vi "e.gate HighSpeedPort Decode Buffer Variable Header Data.vi"(0 "Data in (binary)":u8[](array[numeric]), 1 "Configuration in":T1, 11 "error in (no error)":errorcluster) -> (3 "Configuration out":T1, 4 "Remaining Data out":u8[](array[numeric]), 15 "error out":errorcluster)   [LabVIEW 2016]
doc: "This VI is used to decode all channel related data from a UDBF coded stream to an array of channel data clusters in the configuration cluster."
uses:
  e.gate Configuration.ctl
  e.gate Channel Data.ctl
  e.gate Data Type.ctl
  e.gate Protocol Type.ctl
  e.gate Module  Data.ctl
  e.gateHSP_DLLhandle.ctl
panel:
  out "ChannelAdditionalDatLen 2":i32
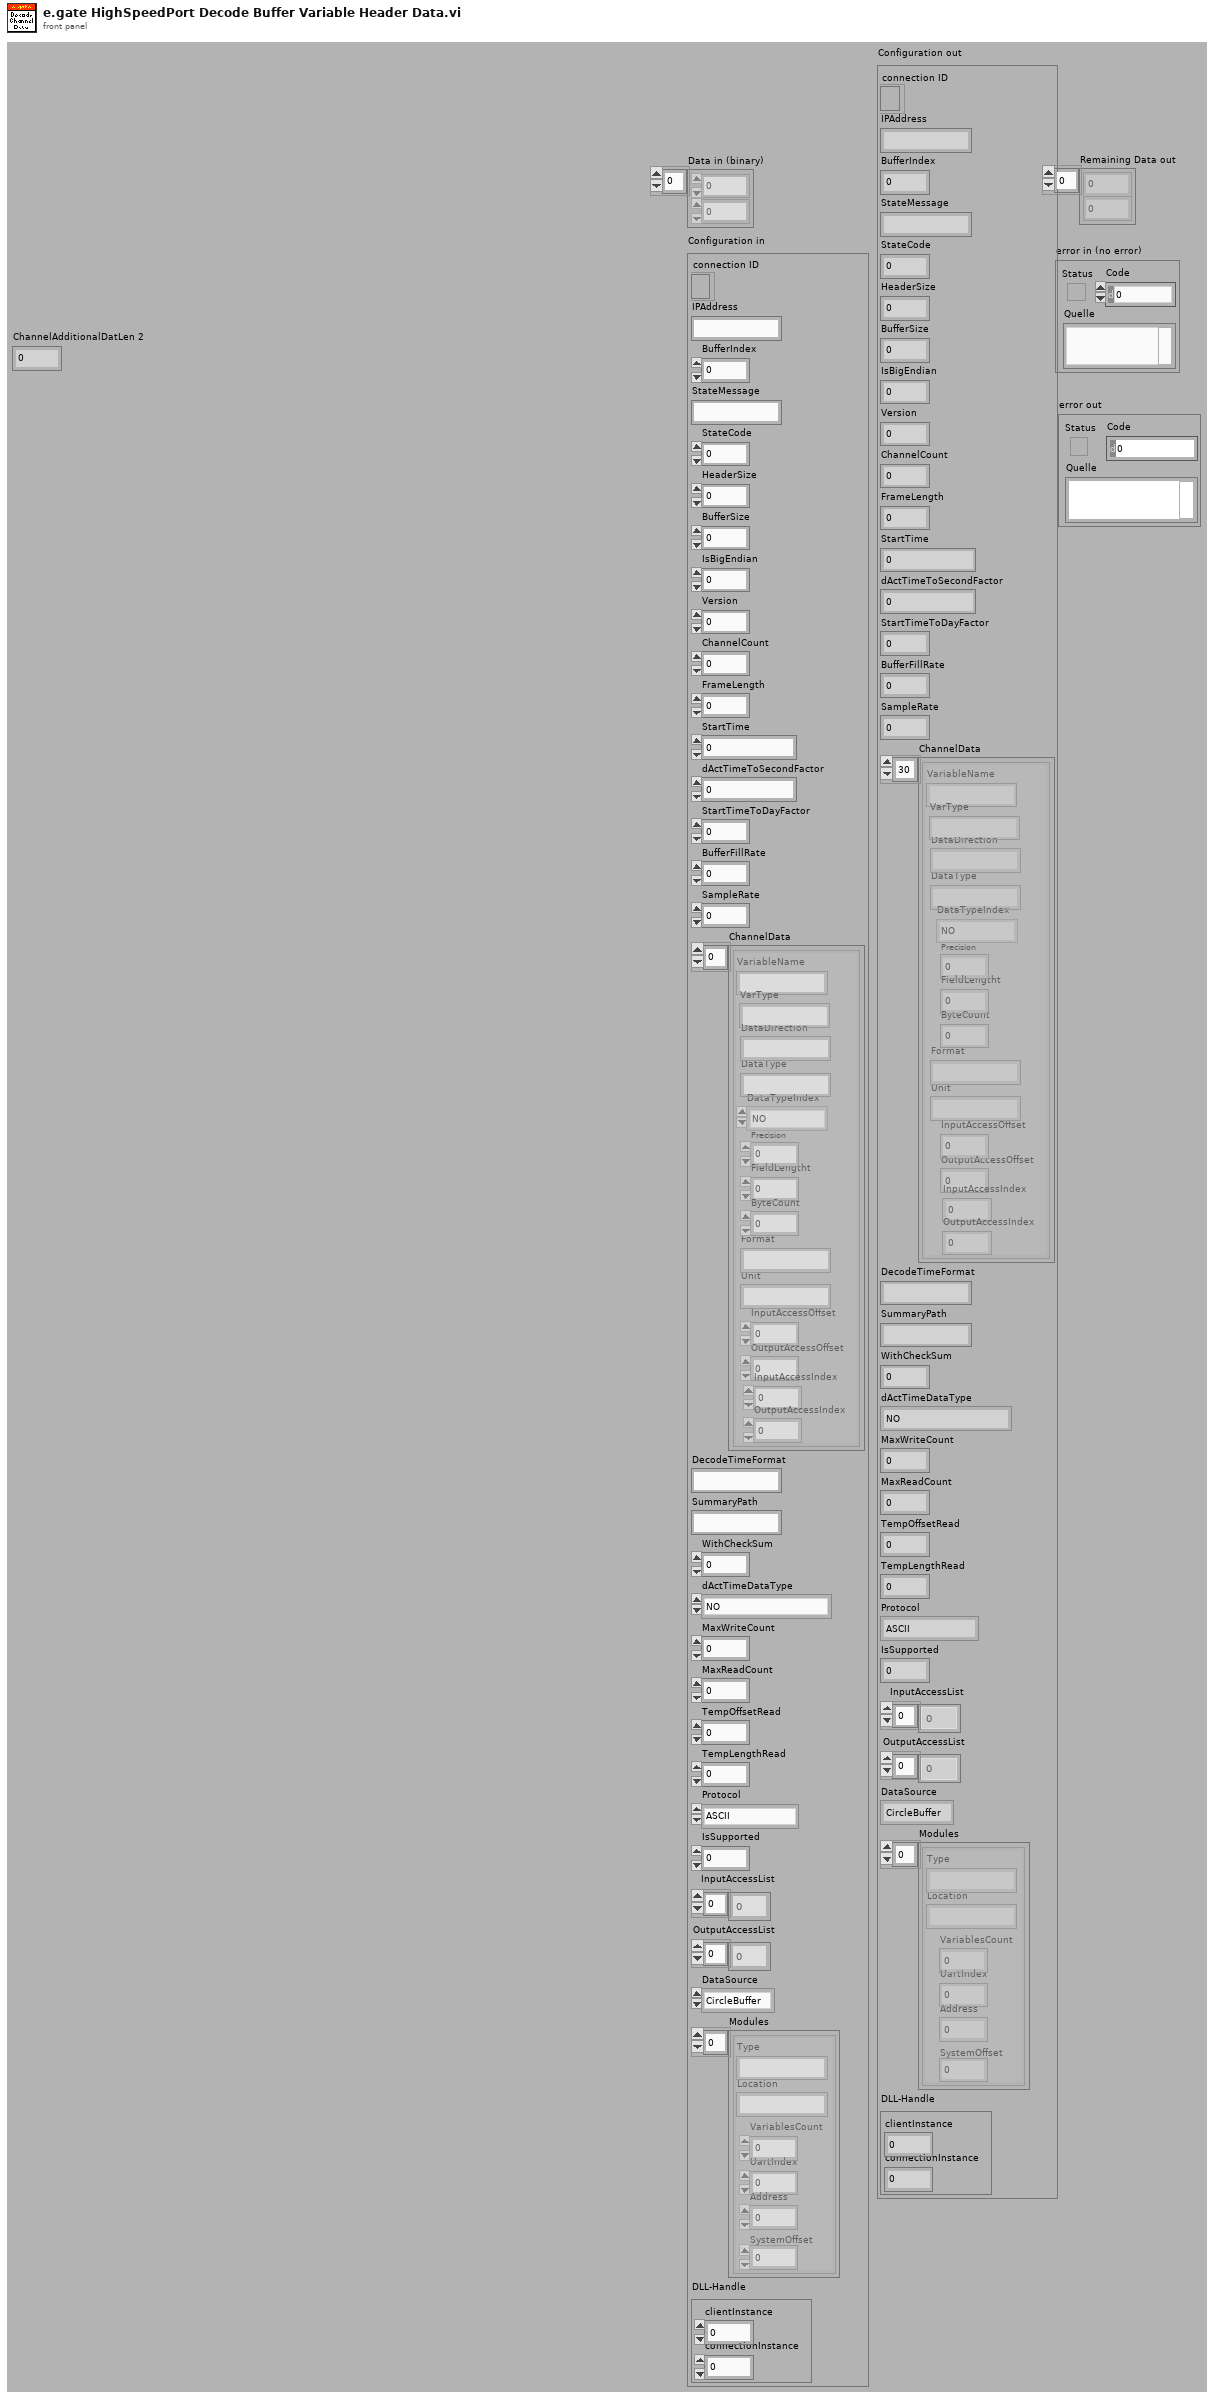
[diagram p1: front panel]
types:
  T1 = typedef "e.gate Configuration.ctl" = cluster{"connection ID":refnum<k5>, "IPAddress":string, "BufferIndex":i32, "StateMessage":string, "StateCode":i8, "HeaderSize":i32, "BufferSize":i32, "IsBigEndian":i32, "Version":i32, "ChannelCount":i32, "FrameLength":i32, "StartTime":dbl, "dActTimeToSecondFactor":dbl, "StartTimeToDayFactor":dbl, "BufferFillRate":dbl, "SampleRate":dbl, "ChannelData":T2[], "DecodeTimeFormat":string, "SummaryPath":string, "WithCheckSum":i32, "dActTimeDataType":T3, "MaxWriteCount":i32, "MaxReadCount":i32, "TempOffsetRead":i32, "TempLengthRead":i32, "Protocol":T4, "IsSupported":i32, "InputAccessList":i32[], "OutputAccessList":i32[], "DataSource":enum16{"CircleBuffer", "test.con Logger", "test.con Archive"}, "Modules":T5[], "DLL-Handle":T6}
  T2 = typedef "e.gate Channel Data.ctl" = cluster{"VariableName":string, "DataDirection":string, "DataType":string, "DataTypeIndex":T3, "Precision":i16, "FieldLengtht":i16, "ByteCount":i32, "Format":string, "Unit":string, "InputAccessOffset":i32, "OutputAccessOffset":i16, "InputAccessIndex":i16, "OutputAccessIndex":i16, "VarType":string}
  T3 = typedef "e.gate Data Type.ctl" = enum16{"NO", "BOOL", "SINT8", "USINT8", "SINT16", "USINT16", "SINT32", "USINT32", "FLOAT", "SET8", "SET16", "SET32", "DOUBLE", "SINT64", "USINT64", "SET64"}
  T4 = typedef "e.gate Protocol Type.ctl" = enum16{"ASCII", "HighspeedPort Online", "HighspeedPort Buffer", "eGateHighspeedPortDLL "}
  T5 = typedef "e.gate Module  Data.ctl" = cluster{"Type":string, "Location":string, "VariablesCount":i16, "UartIndex":i16, "Address":i16, "SystemOffset":i16}
  T6 = typedef "e.gateHSP_DLLhandle.ctl" = cluster{"clientInstance":i32, "connectionInstance":i32}
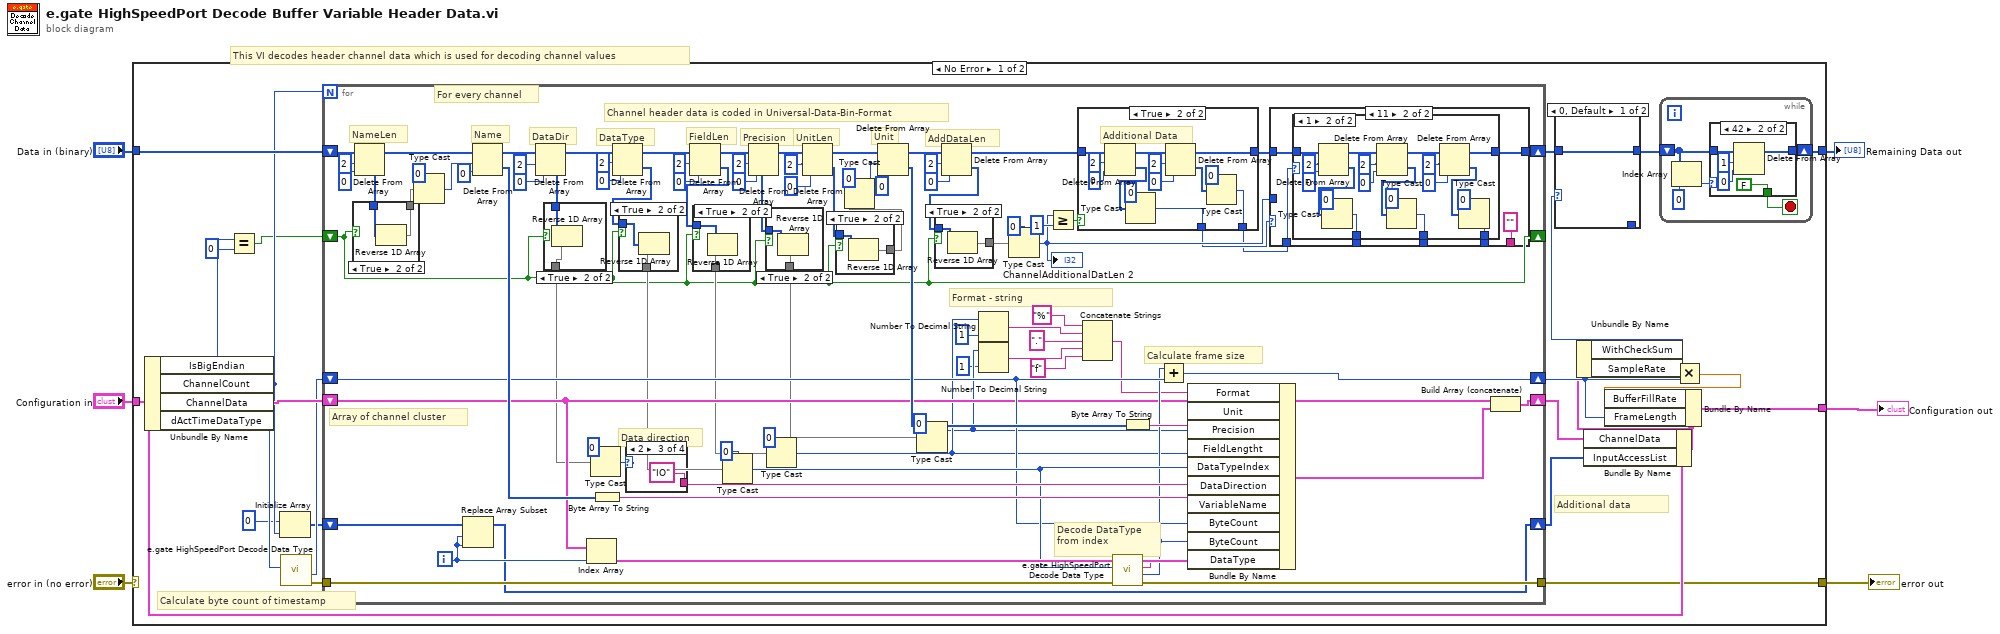
[diagram p0: block diagram]
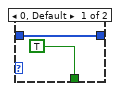
[diagram p2: hidden frame]
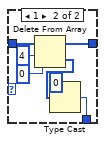
[diagram p3: hidden frame]
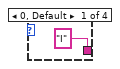
[diagram p11: hidden frame]
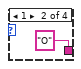
[diagram p12: hidden frame]
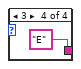
[diagram p13: hidden frame]
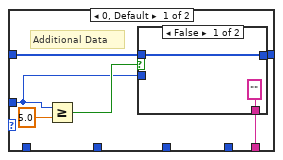
[diagram p14: hidden frame]
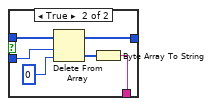
[diagram p15: hidden frame]
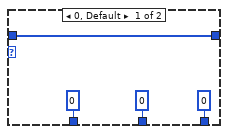
[diagram p16: hidden frame]
diagram:
  # "This VI decodes header channel data which is used for decoding channel values"
  n1 = case shown="No Error" "error in (no error)" {
    selector: "error in (no error)" -> [_ w222]
    tunnel: "Data in (binary)" -> [w30 _]
    tunnel: "Configuration in" -> [w26 w221]
    tunnel: [w24 w222] -> w4
    tunnel: [w23 w221] -> w2
    tunnel: [w18 _] -> w1
    frame No Error {
      # "Additional data"
      # "Calculate byte count of timestamp"
      n2 = Unbundle By Name(w26) -> ("IsBigEndian"=w9:i32, "ChannelCount"=w13:i32, "ChannelData"=w29:T2[], "dActTimeDataType"=w14:T3)
      n3 = Equal?(x=w9, y=0) -> (x = y?=w7:bool)
      n4 = Initialize Array(0 ("Element"), w13) -> (w11:i32[])
      n5 = call "e.gate HighSpeedPort Decode Data Type.vi"("DataTypeIndex"=w14) -> ("error out"=w27:errorcluster, "ByteCount"=w28:i32)  [unwired: 3 in, 6 out]
      n6 = for {
        N: w13 -> [_]
        shift-right: [w105] -> w16
        shift-left: w30 -> [w137]
        shift-right: [w101] -> w22
        shift-left: w28 -> [w86]
        tunnel: w27 -> [w88]
        shift-right: [w81] -> w25
        shift-left: w29 -> [w82]
        tunnel: [w87] -> w24
        shift-right: [w66] -> w10
        shift-left: w11 -> [w68]
        shift-right: [w51] -> _
        shift-left: w7 -> [w51]
        i -> [w67]
        # "AddDataLen"
        # "Unit"
        # "UnitLen"
        # "Precision"
        # "FieldLen"
        # "DataType"
        # "DataDir"
        # "Name"
        # "NameLen"
        # "Decode DataType\nfrom index"
        # "Array of channel cluster"
        # "Calculate frame size"
        # "Data direction"
        # "Format - string"
        # "Channel header data is coded in Universal-Data-Bin-Format"
        # "For every channel"
        n7 = Delete From Array(array=w137, length=2 ("Länge"), index=0 ("Index")) -> (deleted portion=w65:u8[], array with subset deleted=w136:u8[])
        n8 = case shown="True" w51 {
          tunnel: w65 -> [w156 w158]
          tunnel: [w156 w157] -> w64
          frame False {
          }
          frame True {
            n9 = Reverse 1D Array(array=w158) -> (reversed array=w157:u8[])
          }
        }
        n10 = Type Cast(type=i16 0, x=w64) -> (*(type *) &x=w103:i16)
        n11 = Replace Array Subset(array=w68, new element=w67, index=w67) -> (w66:i32[])
        n12 = Delete From Array(array=w136, length=w103, index=0 ("Index")) -> (deleted portion=w99:u8[], array with subset deleted=w135:u8[])
        n13 = Delete From Array(array=w135, length=2 ("Länge"), index=0 ("Index")) -> (deleted portion=w63:u8[], array with subset deleted=w134:u8[])
        n14 = case shown="True" w51 {
          tunnel: w63 -> [w153 w155]
          tunnel: [w153 w154] -> w62
          frame False {
          }
          frame True {
            n15 = Reverse 1D Array(array=w155) -> (reversed array=w154:u8[])
          }
        }
        n16 = Index Array(array=w82, index=w67) -> (element=w100:T2)
        n17 = Type Cast(type=i16 0, x=w62) -> (*(type *) &x=w97:i16)
        n18 = Byte Array To String(unsigned byte array=w99) -> (string=w98:string)
        n19 = Delete From Array(array=w134, length=2 ("Länge"), index=0 ("Index")) -> (deleted portion=w61:u8[], array with subset deleted=w133:u8[])
        n20 = case shown="True" w51 {
          tunnel: w61 -> [w150 w152]
          tunnel: [w150 w151] -> w60
          frame False {
          }
          frame True {
            n21 = Reverse 1D Array(array=w152) -> (reversed array=w151:u8[])
          }
        }
        n22 = case shown="2" w97 {
          tunnel: ["I" "O" "IO" "E"] -> w95
          frame 0, Default {
          }
          frame 1 {
          }
          frame 2 {
          }
          frame 3 {
          }
        }
        n23 = Delete From Array(array=w133, length=2 ("Länge"), index=0 ("Index")) -> (deleted portion=w59:u8[], array with subset deleted=w132:u8[])
        n24 = case shown="True" w51 {
          tunnel: w59 -> [w147 w149]
          tunnel: [w147 w148] -> w58
          frame False {
          }
          frame True {
            n25 = Reverse 1D Array(array=w149) -> (reversed array=w148:u8[])
          }
        }
        n26 = Type Cast(type=i16 0, x=w60) -> (*(type *) &x=w89:i16)
        n27 = Delete From Array(array=w132, length=2 ("Länge"), index=0 ("Index")) -> (deleted portion=w57:u8[], array with subset deleted=w131:u8[])
        n28 = case shown="True" w51 {
          tunnel: w57 -> [w144 w146]
          tunnel: [w144 w145] -> w56
          frame False {
          }
          frame True {
            n29 = Reverse 1D Array(array=w146) -> (reversed array=w145:u8[])
          }
        }
        n30 = Type Cast(type=i16 0, x=w58) -> (*(type *) &x=w76:i16)
        n31 = Delete From Array(array=w131, length=2 ("Länge"), index=0 ("Index")) -> (deleted portion=w55:u8[], array with subset deleted=w130:u8[])
        n32 = case shown="True" w51 {
          tunnel: w55 -> [w141 w143]
          tunnel: [w141 w142] -> w54
          frame False {
          }
          frame True {
            n33 = Reverse 1D Array(array=w143) -> (reversed array=w142:u8[])
          }
        }
        n34 = Type Cast(type=i16 0, x=w54) -> (*(type *) &x=w113:i16)
        n35 = Delete From Array(array=w130, length=w113, index=0 ("Index")) -> (deleted portion=w91:u8[], array with subset deleted=w129:u8[])
        n36 = Type Cast(type=i16 0, x=w56) -> (*(type *) &x=w75:i16)
        n37 = Delete From Array(array=w129, length=2 ("Länge"), index=0 ("Index")) -> (deleted portion=w52:u8[], array with subset deleted=w104:u8[])
        n38 = case shown="True" w51 {
          tunnel: w52 -> [w138 w140]
          tunnel: [w138 w139] -> w53
          frame False {
          }
          frame True {
            n39 = Reverse 1D Array(array=w140) -> (reversed array=w139:u8[])
          }
        }
        n40 = Number To Decimal String(number=w76, width (-)=i16 1 ("Breite (-)")) -> (decimal integer string=w71:string)
        n41 = Number To Decimal String(number=w75, width (-)=i16 1 ("Breite (-)")) -> (decimal integer string=w72:string)
        n42 = Type Cast(type=0, x=w53) -> (*(type *) &x=w102:i32)
        "ChannelAdditionalDatLen 2" <- w102
        n43 = Greater Or Equal?(x=w102, y=1) -> (x >= y?=w107:bool)
        n44 = case shown="True" w107 {
          tunnel: w104 -> [w207 w220]
          tunnel: [w207 w218] -> w106
          tunnel: [_ w211] -> w85
          tunnel: [_ w209] -> w84
          frame False {
          }
          frame True {
            # "Additional Data"
            n45 = Delete From Array(array=w220, length=2 ("Länge"), index=0 ("Index")) -> (deleted portion=w212:u8[], array with subset deleted=w219:u8[])
            n46 = Type Cast(type=0, x=w212) -> (*(type *) &x=w211:i32)
            n47 = Delete From Array(array=w219, length=2 ("Länge"), index=0 ("Index")) -> (deleted portion=w208:u8[], array with subset deleted=w218:u8[])
            n48 = Type Cast(type=0, x=w208) -> (*(type *) &x=w209:i32)
          }
        }
        n49 = Concatenate Strings("%" ("String"), w71, "." ("String"), w72, "f" ("String")) -> (w70:string)
        n50 = call "e.gate HighSpeedPort Decode Data Type.vi"("error in (no errro)"=w88, "DataTypeIndex"=w89) -> ("error out"=w87:errorcluster, "ByteCount"=w83:i32, "DataType"=w80:string)  [unwired: 2 in, 5 out]
        n51 = Byte Array To String(unsigned byte array=w91) -> (string=w90:string)
        n52 = Add(x=w83, y=w86) -> (x+y=w101:i32)
        n53 = Bundle By Name(cluster=w100, "Format"=w70, "Unit"=w90, "Precision"=w75, "FieldLengtht"=w76, "DataTypeIndex"=w89, "DataDirection"=w95, "VariableName"=w98, "ByteCount"=w86, "ByteCount"=w83, "DataType"=w80) -> (w69:T2)
        n54 = case shown="11" w85 {
          tunnel: w106 -> [w168 w183]
          tunnel: [w167 w182] -> w105
          tunnel: w102 -> [w164 _]
          tunnel: w84 -> [_ w181]
          tunnel: [w163 "" ("string")] -> _
          tunnel: [_ w180] -> _
          tunnel: [_ w179] -> _
          tunnel: [_ w178] -> _
          frame 0, Default {
            # "Additional Data"
            n55 = Greater Or Equal?(x=w164, y=5.0) -> (x >= y?=w165:bool)
            n56 = case shown="False" w165 {
              tunnel: w168 -> [w170 w174]
              tunnel: [w170 w173] -> w167
              tunnel: w164 -> [_ w176]
              tunnel: ["" ("string") w171] -> w163
              frame False {
              }
              frame True {
                n57 = Delete From Array(array=w174, length=w176, index=0 ("Index")) -> (deleted portion=w172:u8[], array with subset deleted=w173:u8[])
                n58 = Byte Array To String(unsigned byte array=w172) -> (string=w171:string)
              }
            }
          }
          frame 11 {
            n59 = case shown="1" w181 {
              tunnel: w183 -> [w187 w206]
              tunnel: [w187 w197] -> w182
              tunnel: [0 w190] -> w180
              tunnel: [0 w189] -> w179
              tunnel: [0 w188] -> w178
              frame 0, Default {
              }
              frame 1 {
                n60 = Delete From Array(array=w206, length=2 ("Länge"), index=0 ("Index")) -> (deleted portion=w195:u8[], array with subset deleted=w203:u8[])
                n61 = Type Cast(type=0, x=w195) -> (*(type *) &x=w190:i32)
                n62 = Delete From Array(array=w203, length=2 ("Länge"), index=0 ("Index")) -> (deleted portion=w193:u8[], array with subset deleted=w202:u8[])
                n63 = Type Cast(type=0, x=w193) -> (*(type *) &x=w189:i32)
                n64 = Delete From Array(array=w202, length=2 ("Länge"), index=0 ("Index")) -> (deleted portion=w191:u8[], array with subset deleted=w197:u8[])
                n65 = Type Cast(type=0, x=w191) -> (*(type *) &x=w188:i32)
              }
            }
          }
        }
        n66 = Build Array (concatenate)(w82, w69) -> (w81:T2[])
      }
      n67 = Bundle By Name(cluster=w26, "ChannelData"=w25, "InputAccessList"=w10) -> (w19:T1)
      n68 = Unbundle By Name(w19) -> ("WithCheckSum"=w17:i32, "SampleRate"=w21:dbl)
      n69 = case shown="0, Default" w17 {
        tunnel: w16 -> [w43 w50]
        tunnel: [w43 w49] -> w15
        tunnel: [_ w44] -> _
        frame 0, Default {
        }
        frame 1 {
          n70 = Delete From Array(array=w50, length=4, index=0) -> (deleted portion=w46:u8[], array with subset deleted=w49:u8[])
          n71 = Type Cast(type=0, x=w46) -> (*(type *) &x=w44:i32)
        }
      }
      n72 = while {
        shift-right: [w35] -> w18
        shift-left: w15 -> [w32]
        stop <- w34 stop-if-true
        n73 = Index Array(array=w32, index=0 ("Index")) -> (element=w31:u8)
        n74 = case shown="42" w31 {
          tunnel: w32 -> [w37 w42]
          tunnel: [w37 w39] -> w35
          tunnel: [TRUE ("Stopp") FALSE ("Stopp")] -> w34
          frame 0, Default {
          }
          frame 42 {
            n75 = Delete From Array(array=w42, length=1 ("Länge"), index=0 ("Index")) -> (array with subset deleted=w39:u8[])  [unwired: 1 out]
          }
        }
      }
      n76 = Multiply(x=w21, y=w22) -> (x*y=w20:dbl)
      n77 = Bundle By Name(cluster=w19, "BufferFillRate"=w20, "FrameLength"=w22) -> (w23:T1)
    }
    frame Error {
    }
  }
  "error out" <- w4
  "Configuration out" <- w2
  "Remaining Data out" <- w1
